vi "GlobalHopper.vi"() -> ()   [LabVIEW 2020]
panel:
  out "OUT_Photon_Cannons_On":bool
  out "OUT_Hopper_Disallow_States":bool
  out "OUT_Auto_Stow_From_Hopper":bool
  out "OUT_Hopper_Arm_Position":bool
  out "OUT_Hopper_Extended":bool
  out "SEN_Beam_Break_Center":bool
  out "REF_Hopper_Beam_Break_Center":string
  out "REF_Hopper_Wings":string
  # "DEVICE REFERENCE NAMES"
  # "CONSTANTS"
  # "DRIVER STATION DATA"
  # "SENSORS"
  # "OUTPUTS"
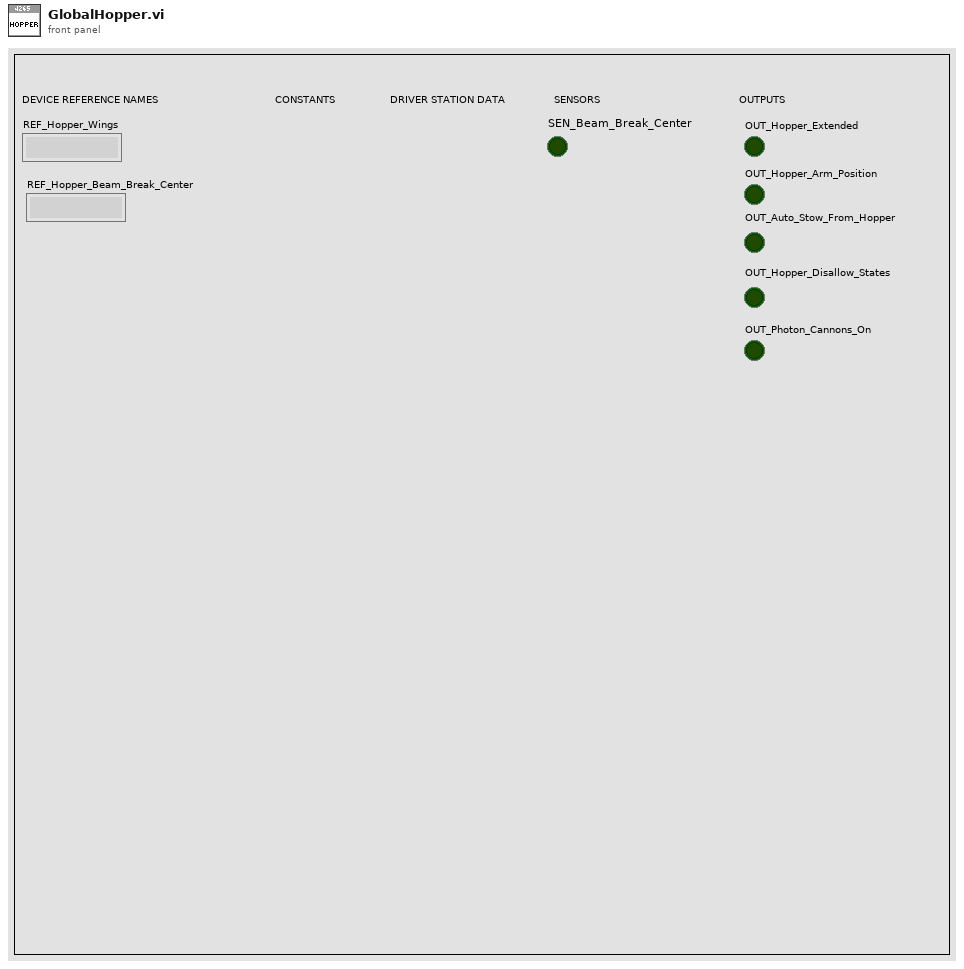
[diagram p1: front panel]
diagram:
